vi "Get Subscription Topics.vi"() -> (2 "Topic Subscriptions":T1[](array[typedef]))   [LabVIEW 2021, in "MQTT Bridge.lvlib"]
uses:
  <vilib>/LabVIEW Open Source Project/MQTT Control Packets/Control Packets/SUBSCRIBE/Topic Subscription -- cluster.ctl
  <vilib>/LabVIEW Open Source Project/MQTT Control Packets/Control Packets/ControlPacket/QualityOfService -- enum.ctl
  MQTT Bridge.lvlib
  <vilib>/LabVIEW Open Source Project/MQTT Control Packets/Control Packets/ControlPacket/ControlPacket.lvclass
  <vilib>/LabVIEW Open Source Project/MQTT Control Packets/Control Packets/SUBSCRIBE/SUBSCRIBE.lvclass
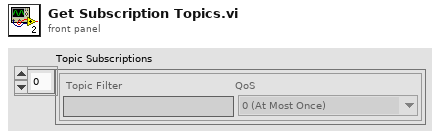
[diagram p1: front panel]
types:
  T1 = typedef "MQTT_Control_Packets.lvlib/SUBSCRIBE.lvclass/Topic Subscription -- cluster.ctl" = cluster{"Topic Filter":string, "QoS":T2}
  T2 = typedef "MQTT_Control_Packets.lvlib/ControlPacket.lvclass/QualityOfService -- enum.ctl" = enum16{"0 (At Most Once)", "1 (At Least Once)", "2 (Exactly Once)"}
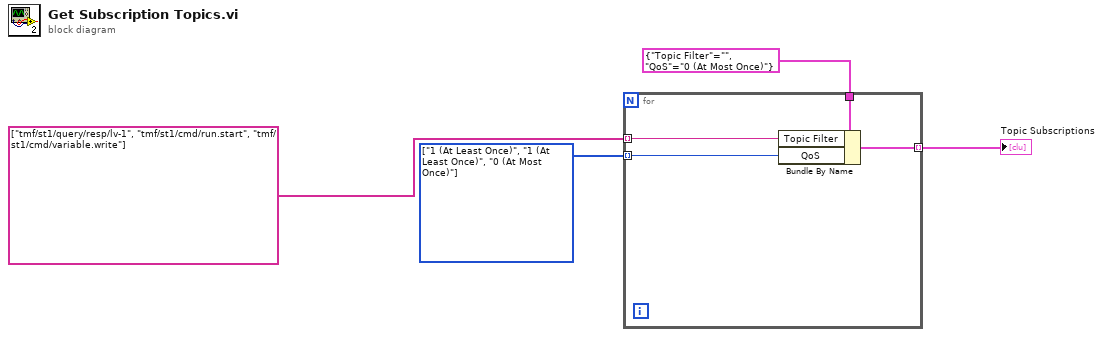
[diagram p0: block diagram]
diagram:
  w1 = T2[] [enum."1 (At Least Once)", enum."1 (At Least Once)", enum."0 (At Most Once)"] items=["0 (At Most Once)", "1 (At Least Once)", "2 (Exactly Once)"] ("Array")
  n1 = for {
    tunnel: [w8] -> w4 mode=indexing
    tunnel: T1 {"Topic Filter"="", "QoS"=enum."0 (At Most Once)"} ("Topic Subscription") -> [w7]
    tunnel: string[] ["tmf/st1/query/resp/lv-1", "tmf/st1/cmd/run.start", "tmf/st1/cmd/variable.write"] ("Topic Filter") -> [w6] mode=indexing
    tunnel: w1 -> [w5] mode=indexing
    n2 = Bundle By Name(cluster=w7, "Topic Filter"=w6, "QoS"=w5) -> (w8:T1)
  }
  "Topic Subscriptions" <- w4
